vi "LabVIEW Interface MAIN.vi"() -> ()   [LabVIEW 2018]
uses:
  src/geve-monitoring_data_cluster.ctl
  <vilib>/Instr/_visa.llb/VISA Configure Serial Port (Instr).vi
panel:
  out "title":string
  in  "Stop":bool
  out "Motor Position":dbl
  out "Plateau Pressure":dbl
  out "Pressure":dbl
  out "Mixed Signal Graph":cluster{timestamp[], dbl[]}[](graph)
  out "BPM":dbl
  out "PEEP":dbl
  out "Tidal Volume":dbl
  out "IE Ratio":dbl
  out "LOG":string[](array[string])
  out "INITIALISATION ERROR":bool
  out "HIGH PRESSURE":bool
  out "LOW PRESSURE":bool
  # "LATEST VALUE"
  # "Motor Position"
  # "Plateau Pressure"
  # "Pressure"
  # "LIVE DATA"
  # "POTENTIOMETERS SETTINGS"
  # "BPM"
  # "PEEP"
  # "IE RATIO"
  # "TIDAL VOLUME"
  # "LOG"
  # "ALARMS"
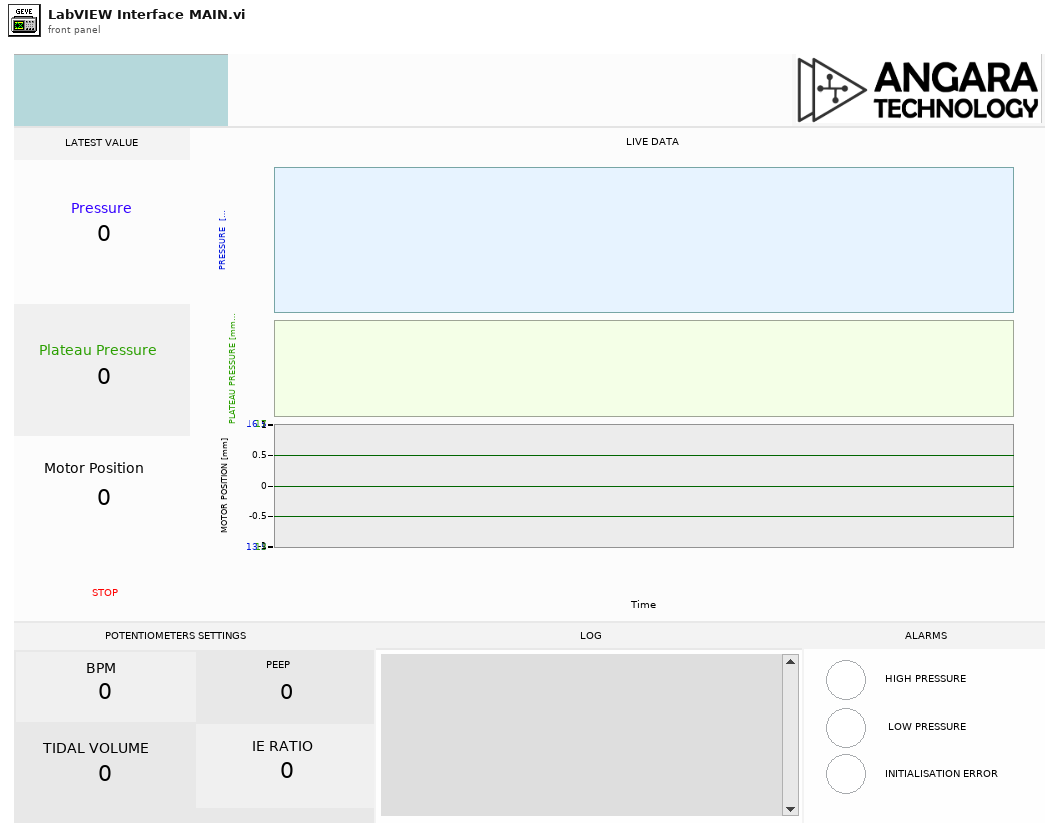
[diagram p1: front panel]
types:
  T1 = typedef "geve-monitoring_data_cluster.ctl" = cluster{"On/Off":bool, "Error Ack":bool, "bpm":dbl, "VT":dbl, "IE":dbl, "PEEP":dbl, "Pressure":dbl, "Plateau Pressure":dbl, "Motor Position":dbl, "Alarm P High":bool, "Alarm P Low":bool, "Alarm Init":bool}
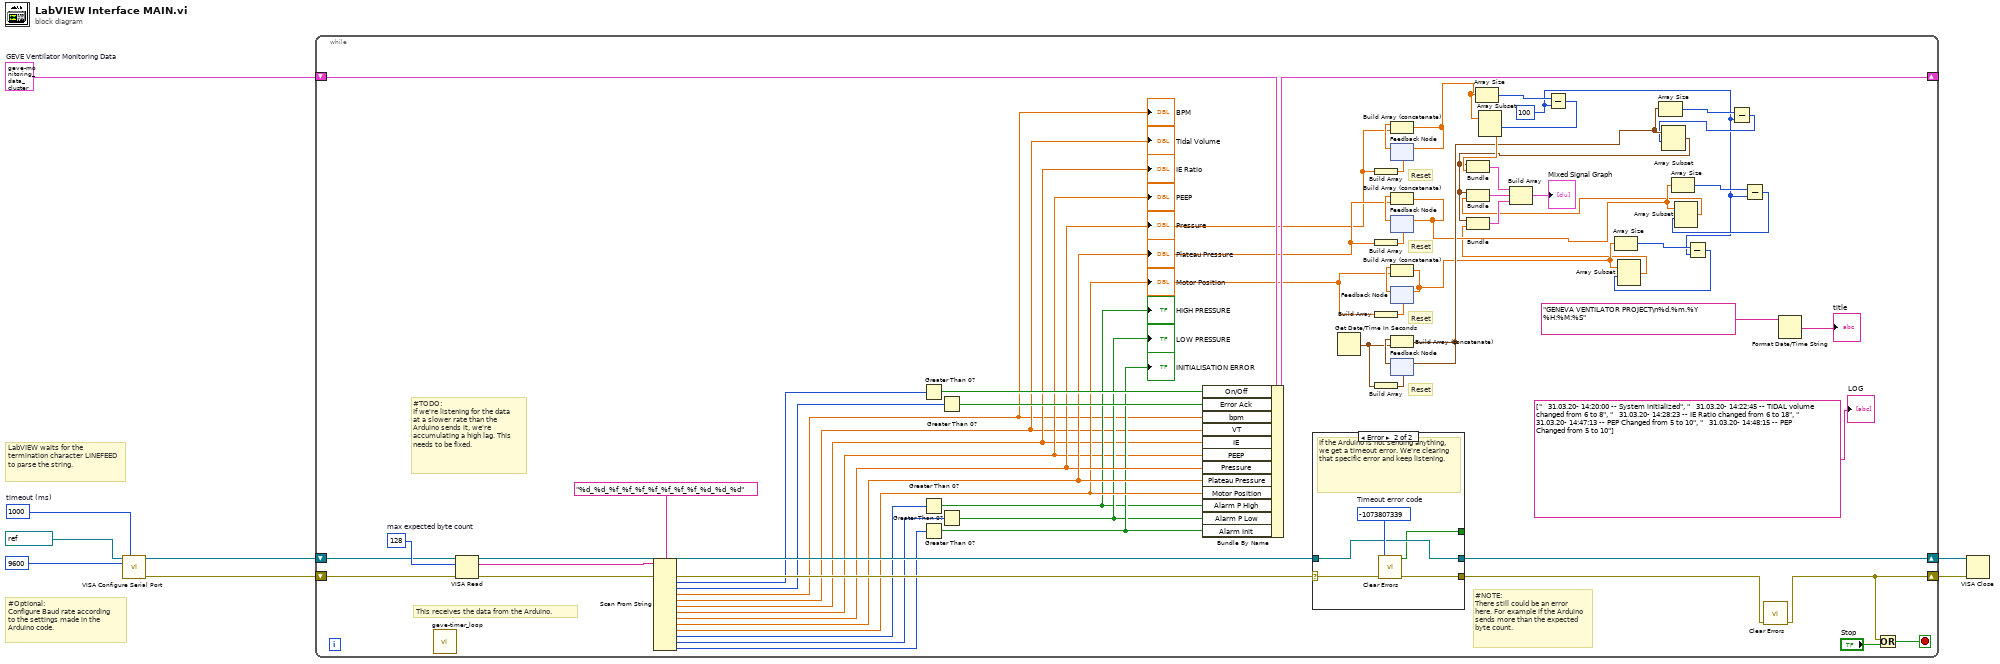
[diagram p0: block diagram]
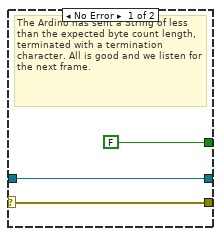
[diagram p2: hidden frame]
diagram:
  w2 = T1 {"On/Off"=FALSE, "Error Ack"=FALSE, "bpm"=0.0, "VT"=0.0, "IE"=0.0, "PEEP"=0.0, "Pressure"=0.0, "Plateau Pressure"=0.0, "Motor Position"=0.0, "Alarm P High"=FALSE, "Alarm P Low"=FALSE, "Alarm Init"=FALSE}  # GEVE Ventilator Monitoring Data
  w4 = u32 1000  # timeout (ms)
  # "#Optional:\nConfigure Baud rate according to the settings made in the Arduino code."
  # "LabVIEW waits for the termination character LINEFEED to parse the string."
  n1 = call-poly "VISA Configure Serial Port"("VISA resource name"=refnum<visa-resource-name> "COM4", "timeout (10sec)"=w4, "baud rate (9600)"=u32 9600) -> ("VISA resource name out"=w8:refnum<visa-resource-name>, "error out"=w6:errorcluster)  [unwired: 11 in]
  n2 = while {
    shift-right: [w57] -> w7
    shift-left: w8 -> [w66]
    shift-right: [w9] -> w5
    shift-left: w6 -> [w65]
    shift-right: [w62] -> _
    shift-left: w2 -> [w63]
    stop <- w72 stop-if-true
    w11 = 100 ("y")
    w71 = u32 128  # max expected byte count
    # "Reset"
    # "Reset"
    # "Reset"
    # "Reset"
    # "#TODO:\nIf we're listening for the data at a slower rate than the Arduino sends it, we're accumulating a high lag. This needs to be fixed."
    # "This receives the data from the Arduino."
    # "#NOTE:\nThere still could be an error here. For example if the Arduino sends more than the expected byte count."
    n3 = call "geve-timer_loop.vi"() -> ()  [unwired: 11 in, 1 out]
    n4 = VISA Read(VISA resource name=w66, byte count=w71, error in (no error)=w65) -> (VISA resource name out=w70:refnum<visa-resource-name>, read buffer=w68:string, error out=w67:errorcluster)  [unwired: 1 out]
    n5 = Scan From String(format string="%d_%d_%f_%f_%f_%f_%f_%f_%f_%d_%d_%d", input string=w68, error in=w67) -> (error out=w69:errorcluster, output 1=w61:i32, output 2=w60:i32, output 3=w28:dbl, output 4=w29:dbl, output 5=w30:dbl, output 6=w31:dbl, output 7=w42:dbl, output 8=w45:dbl, output 9=w35:dbl, output 10=w36:i32, output 11=w37:i32, output 12=w38:i32)  [unwired: 13 in, 2 out]
    "BPM" <- w28
    "Tidal Volume" <- w29
    "PEEP" <- w31
    "IE Ratio" <- w30
    "Pressure" <- w42
    "Plateau Pressure" <- w45
    "Motor Position" <- w35
    n6 = Greater Than 0?(x=w61) -> (x > 0?=w59:bool)
    n7 = Greater Than 0?(x=w36) -> (x > 0?=w32:bool)
    "HIGH PRESSURE" <- w32
    n8 = Greater Than 0?(x=w38) -> (x > 0?=w34:bool)
    "INITIALISATION ERROR" <- w34
    n9 = Greater Than 0?(x=w60) -> (x > 0?=w58:bool)
    n10 = Greater Than 0?(x=w37) -> (x > 0?=w33:bool)
    "LOW PRESSURE" <- w33
    n11 = Bundle By Name(cluster=w63, "On/Off"=w59, "Error Ack"=w58, "bpm"=w28, "VT"=w29, "IE"=w30, "PEEP"=w31, "Pressure"=w42, "Plateau Pressure"=w45, "Motor Position"=w35, "Alarm P High"=w32, "Alarm P Low"=w33, "Alarm Init"=w34) -> (w62:T1)
    n12 = case shown="Error" w69 {
      selector: w69 -> [w76 w81]
      tunnel: [w76 w79] -> w10
      tunnel: [w75 w78] -> w57
      tunnel: w70 -> [w75 w78]
      tunnel: [FALSE ("specific error cleared?") w77] -> _
      frame No Error {
        # "The Ardino has sent a String of less than the expected byte count length, terminated with a termination character. All is good and we listen for the next frame."
      }
      frame Error {
        w80 = -1073807339  # Timeout error code
        # "If the Arduino is not sending anything, we get a timeout error. We're clearing that specific error and keep listening."
        n13 = call <vilib>:"Clear Errors.vi"("error in (no error)"=w81, "specific error code to clear (0: all)"=w80) -> ("error out"=w79:errorcluster, "specific error cleared?"=w77:bool)  [unwired: 4 in]
      }
    }
    n14 = Get Date/Time In Seconds() -> (seconds since 1Jan1904=w49:timestamp)
    n15 = Build Array(w42) -> (w43:dbl[])
    n16 = Build Array(w45) -> (w47:dbl[])
    n17 = Build Array(w35) -> (w41:dbl[])
    n18 = Build Array(w49) -> (w48:timestamp[])
    n19 = feedback #1(w43) -> (w44:dbl[])
    n20 = Build Array (concatenate)(w44, w42) -> (w22:dbl[])
    n21 = feedback-in #1(w22) -> ()
    n22 = feedback #2(w47) -> (w46:dbl[])
    n23 = Build Array (concatenate)(w46, w45) -> (w17:dbl[])
    n24 = feedback-in #2(w17) -> ()
    n25 = feedback #3(w41) -> (w40:dbl[])
    n26 = Build Array (concatenate)(w40, w35) -> (w18:dbl[])
    n27 = feedback-in #3(w18) -> ()
    n28 = feedback #4(w48) -> (w50:timestamp[])
    n29 = Build Array (concatenate)(w50, w49) -> (w21:timestamp[])
    n30 = feedback-in #4(w21) -> ()
    n31 = Array Size(array=w22) -> (size(s)=w27:i32)
    n32 = Subtract(x=w27, y=w11) -> (x-y=w26:i32)
    n33 = Array Subset(array=w22, index=w26) -> (w25:dbl[])  [unwired: 1 in]
    n34 = Array Size(array=w18) -> (size(s)=w23:i32)
    n35 = Array Size(array=w21) -> (size(s)=w24:i32)
    n36 = Array Size(array=w17) -> (size(s)=w12:i32)
    n37 = Subtract(x=w23, y=w11) -> (x-y=w16:i32)
    n38 = Array Subset(array=w18, index=w16) -> (w13:dbl[])  [unwired: 1 in]
    n39 = Subtract(x=w24, y=w11) -> (x-y=w20:i32)
    n40 = Array Subset(array=w21, index=w20) -> (w15:timestamp[])  [unwired: 1 in]
    n41 = Bundle(w15, w25) -> (w53:cluster{timestamp[], dbl[]})  [unwired: 1 in]
    n42 = Bundle(w15, w13) -> (w51:cluster{timestamp[], dbl[]})  [unwired: 1 in]
    n43 = Subtract(x=w12, y=w11) -> (x-y=w19:i32)
    n44 = Array Subset(array=w17, index=w19) -> (w14:dbl[])  [unwired: 1 in]
    n45 = Bundle(w15, w14) -> (w52:cluster{timestamp[], dbl[]})  [unwired: 1 in]
    n46 = Build Array(w53, w52, w51) -> (→"Mixed Signal Graph":cluster{timestamp[], dbl[]}[])
    n47 = call <vilib>:"Clear Errors.vi"("error in (no error)"=w10) -> ("error out"=w9:errorcluster)  [unwired: 5 in, 1 out]
    n48 = Format Date/Time String(time format string (%c)="GENEVA VENTILATOR PROJECT\n%d.%m.%Y      %H:%M:%S") -> (date/time string=→"title":string)  [unwired: 2 in]
    n49 = Or(x=w9, y="Stop") -> (x .or. y?=w72:bool)
    "LOG" <- string[] ["   31.03.20- 14:20:00 -- System initialized", "   31.03.20- 14:22:45 -- TIDAL volume changed from 6 to 8", "   31.03.20- 14:28:23 -- IE Ratio changed from 6 to 18", "   31.03.20- 14:47:13 -- PEP Changed from 5 to 10", "   31.03.20- 14:48:15 -- PEP Changed from 5 to 10"] ("LOG")
  }
  n50 = VISA Close(VISA resource name=w7, error in (no error)=w5) -> ()  [unwired: 1 out]
